vi "Filter Items.vi"(10 "Names":string[](array[string]), 11 "Filter":string) -> (2 "Filtered Names":string[](array[string]))   [LabVIEW 2020, in "Linker Info.lvlib"]
uses:
  Linker Info.lvlib
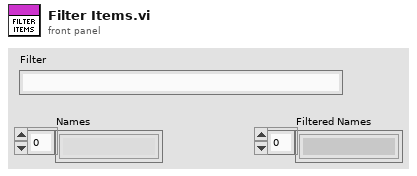
[diagram p1: front panel]
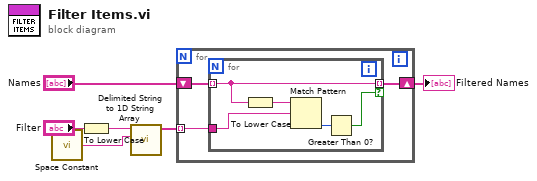
[diagram p0: block diagram]
diagram:
  n1 = call <vilib>:"Space Constant.vi"() -> ("String"=w5:string)
  n2 = To Lower Case(string="Filter") -> (all lower case string=w2:string)
  n3 = call <vilib>:"Delimited String to 1D String Array.vi"("delimiter"=w5, "delimited string"=w2) -> ("string array"=w4:string[])  [unwired: 9 in]
  n4 = for {
    tunnel: w4 -> [w9] mode=indexing
    shift-right: [w7] -> w3
    shift-left: "Names" -> [w8]
    n5 = for {
      tunnel: w9 -> [w14]
      tunnel: w8 -> [w10] mode=indexing
      tunnel: [w10] -> w7 mode=indexing if=w12
      n6 = To Lower Case(string=w10) -> (all lower case string=w11:string)
      n7 = Match Pattern(string=w11, regular expression=w14) -> (offset past match=w13:i32)  [unwired: 1 in, 3 out]
      n8 = Greater Than 0?(x=w13) -> (x > 0?=w12:bool)
    }
  }
  "Filtered Names" <- w3
